vi "CTRE_Phoenix_CANcoder_RefNumRegistrySet.vi"(8 "error in (no error)":errorcluster, 9 "Test Mode Only":bool, 10 "refnum name":string="My CANcoder RefNum", 11 "CTRE_CANcoder_DeviceRef":T1) -> (0 "error out":errorcluster, 3 "CTRE_CANcoder_DeviceRef":T1)   [LabVIEW 2019]
uses:
  <vilib>/Rock Robotics/WPI/Utilities/Refnum Registry Operation.ctl
  <vilib>/Rock Robotics/WPI/ThirdParty/Phoenix-LabVIEW/CANCoder/Controls/CTRE_Phoenix_CANcoder_DeviceRef.ctl
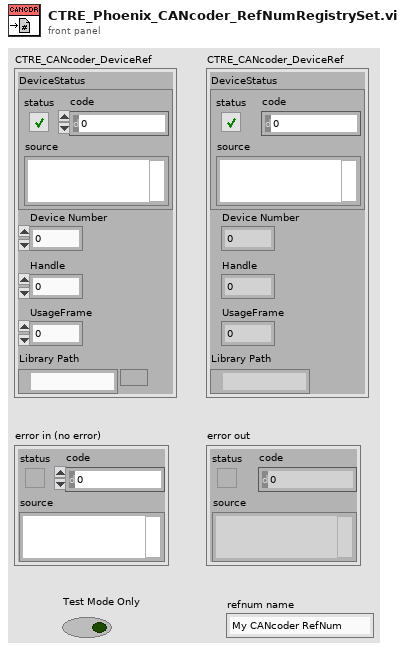
[diagram p1: front panel]
types:
  T1 = typedef "CTRE_Phoenix_CANcoder_DeviceRef.ctl" = cluster{"DeviceStatus":errorcluster, "Device Number":u8, "Handle":u64, "UsageFrame":u32, "Library Path":path}
  T2 = typedef "Refnum Registry Operation.ctl" = enum16{"set", "get", "delete", "get all names", "read name"}
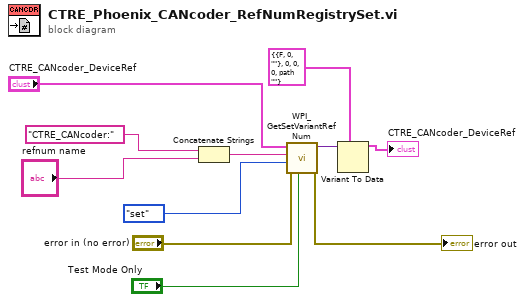
[diagram p0: block diagram]
diagram:
  n1 = Concatenate Strings("CTRE_CANcoder:", "refnum name") -> (w11:string)
  n2 = call <vilib>:"WPI_GetSetVariantRefNum.vi"("Test Mode Only"="Test Mode Only", "error in (no error)"="error in (no error)", "Operation"=Refnum_Registry_Operation."set" ("menu"), "refnum name"=w11, "DevRef"="CTRE_CANcoder_DeviceRef") -> ("error out"=→"error out":errorcluster, "DevRef"=w4:variant)  [unwired: 4 in, 1 out]
  n3 = Variant To Data(type=T1 {"DeviceStatus"={"status"=FALSE, "code"=0, "source"=""}, "Device Number"=0, "Handle"=0, "UsageFrame"=0, "Library Path"=path ""} ("CTRE_CANcoder_DeviceRef"), Variant=w4) -> (data=→"CTRE_CANcoder_DeviceRef":T1)  [unwired: 1 in, 1 out]
